vi "Start Log.vi"(8 "error in (no error)":errorcluster, 10 "tdms file":refnum<k34>, 11 "Acquired Result in":refnum<class "Acquired Result.lvclass">) -> (0 "error out":errorcluster, 2 "tdms file out":refnum<k34>, 3 "Acquired Result out":refnum<class "Acquired Result.lvclass">)   [LabVIEW 2016, in "Acquired Result.lvclass"]
uses:
  Acquired Result.lvclass
  Acquired Result.lvclass/Acquired Result.ctl
  Read Group.vi
  Read Channels.vi
  Read Settings.vi
  Read Time group.vi
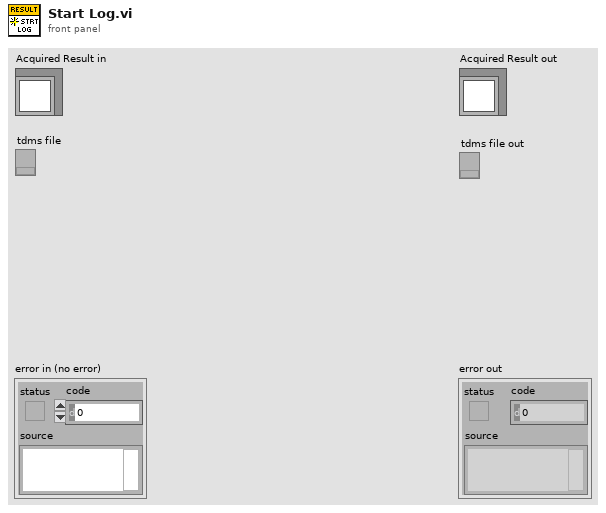
[diagram p1: front panel]
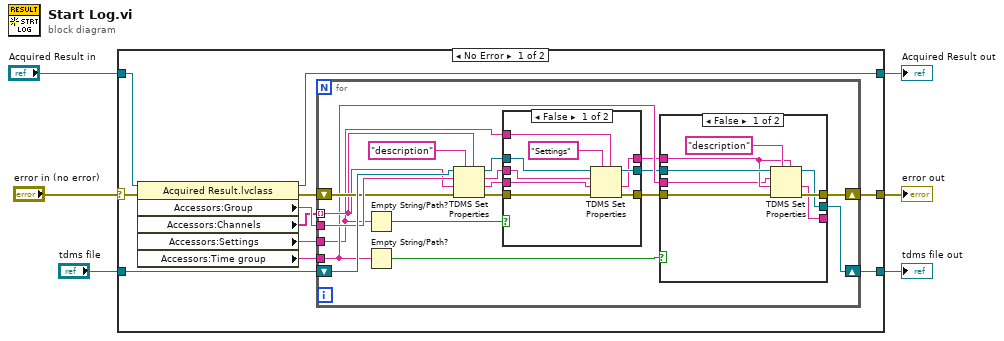
[diagram p0: block diagram]
diagram:
  n1 = case shown="No Error" "error in (no error)" {
    selector: "error in (no error)" -> [w10 w61]
    tunnel: [w16 w61] -> w5
    tunnel: [w11 w60] -> w3
    tunnel: "Acquired Result in" -> [w12 w60]
    tunnel: "tdms file" -> [w14 w59]
    tunnel: [w13 w59] -> w1
    frame No Error {
      n2 = property class="Acquired Result.lvclass"(reference=w12, error in=w10) -> (reference out=w11:refnum<class "Acquired Result.lvclass">, error out=w9:errorcluster, "Accessors:Group"=w17:string, "Accessors:Channels"=w15:string[], "Accessors:Settings"=w8:string, "Accessors:Time group"=w7:string)
      n3 = for {
        tunnel: w17 -> [w34]
        shift-right: [w19] -> w13
        shift-left: w14 -> [w35]
        shift-right: [w20] -> w16
        shift-left: w9 -> [w33]
        tunnel: w15 -> [w30] mode=indexing
        tunnel: w8 -> [w18]
        tunnel: w7 -> [w29]
        n4 = Empty String/Path?(string/path=w18) -> (empty?=w23:bool)
        n5 = Empty String/Path?(string/path=w29) -> (empty?=w31:bool)
        n6 = TDMS Set Properties(5:w30, 7:"description", 8:w33, 9:w30, 10:w34, 11:w35) -> (0:w25:errorcluster, 1:w26:string, 2:w28:string, 3:w27:refnum<k34>)
        n7 = case shown="False" w23 {
          tunnel: w27 -> [w44 w47]
          tunnel: w25 -> [w43 w46]
          tunnel: [w42 w46] -> w21
          tunnel: [w41 w47] -> w22
          tunnel: w26 -> [w39 w45]
          tunnel: w28 -> [w38 _]
          tunnel: [w37 w45] -> w24
          tunnel: w18 -> [w36 _]
          frame False {
            n8 = TDMS Set Properties(5:w36, 7:"Settings", 8:w43, 9:w39, 10:w38, 11:w44) -> (0:w42:errorcluster, 1:w37:string, 3:w41:refnum<k34>)  [unwired: 1 out]
          }
          frame True {
          }
        }
        n9 = case shown="False" w31 {
          tunnel: w22 -> [w55 w58]
          tunnel: w21 -> [w54 w57]
          tunnel: [w53 w57] -> w20
          tunnel: [w52 w58] -> w19
          tunnel: w24 -> [w50 w56]
          tunnel: w29 -> [w49 _]
          tunnel: [w48 w56] -> _
          frame False {
            n10 = TDMS Set Properties(5:w50, 7:"description", 8:w54, 9:w50, 10:w49, 11:w55) -> (0:w53:errorcluster, 1:w48:string, 3:w52:refnum<k34>)  [unwired: 1 out]
          }
          frame True {
          }
        }
      }
    }
    frame Error {
    }
  }
  "error out" <- w5
  "Acquired Result out" <- w3
  "tdms file out" <- w1
